vi "Full Density Matrix Heatmap.vi"(7 "QuWires Array":refnum<class "QuWire.lvclass">) -> ()   [LabVIEW 2020]
uses:
  QuSim/QuWire/QuWire.lvclass
panel:
  out "Real Amplitude":dbl[][](graph)
  out "Imaginary Amplltude":dbl[][](graph)
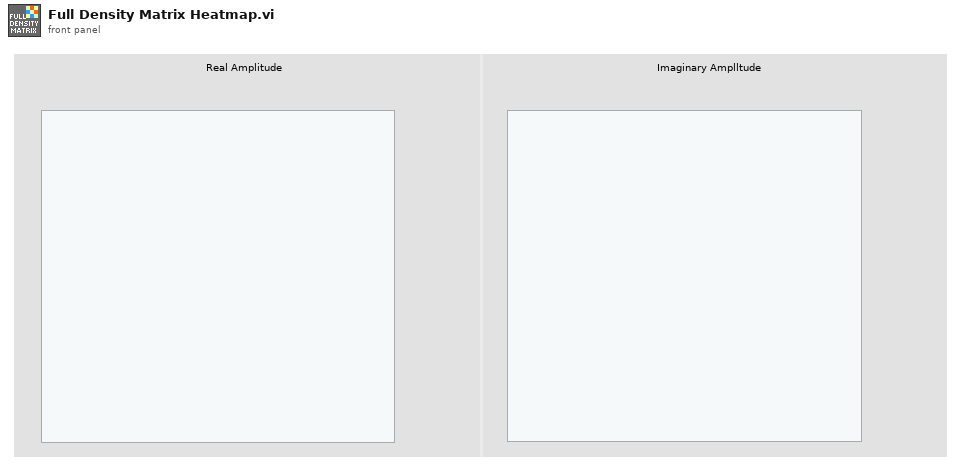
[diagram p1: front panel]
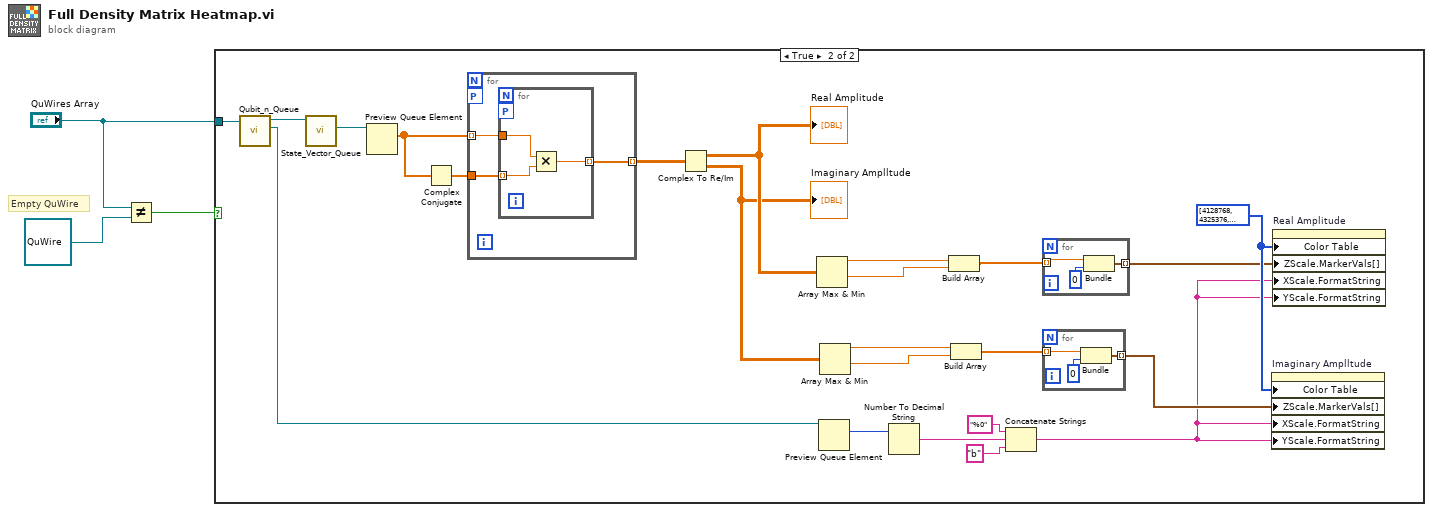
[diagram p0: block diagram]
diagram:
  # "Empty QuWire"
  n1 = Not Equal?(x="QuWires Array", y=refnum<class "QuWire.lvclass"> refnum ("QuWire in")) -> (x != y?=w1:bool)
  n2 = case shown="True" w1 {
    tunnel: "QuWires Array" -> [_ w7]
    frame False {
    }
    frame True {
      w26 = u32[] [4128768, 4325376, 4587520, 4718592, 4915200, 5111808, 5308416, 5505024, 5767168, 5963776, 6160384, 6356992, 6553600, 6750208, 6946816, 7143424, 7340032, 7536640, 7733248, 7929856, 8126464, 8323072, 8519680, 8716288, 8912896, 9109504, 9306112, 9502720, 9699328, 9895936, 10092544, 10289152, 10485760, 10682368, 10878976, 11075584, 11272192, 11468800, 11665408, 11862016, 12058624, 12255232, 12451840, 12648448, 12845056, 13041664, 13238272, 13434880, 13631488, 13828096, 14024704, 14221312, 14417920, 14614528, 14811136, 15007744, 15204352, 15400960, 15597568, 15794176, 16056320, 16187392, 16449536, 16580608, 16711937, 16647683, 16648453, 16649479, 16650250, 16585740, 16586510, 16587536, 16522770, 16523796, 16524566, 16460057, 16461083, 16396317, 16397343, 16398113, 16333604, 16334629, 16335400, 16270634, 16271660, 16272686, 16273713, 16208947, 16209716, 16210743, 16145977, 16147003, 16148029, 16083264, 16084290, 16019523, 16020806, 16021320, 16022602, 15957836, 15958607, 15959633, 15894867, 15896149, 15896663, 15832153, 15833179, 15834205, 15769440, 15770210, 15771236, 15706470, 15707496, 15708522, 15644012, 15644785, 15646076, 15712646, 15713936, 15715226, 15781797, 15783087, 15784377, 15850948, 15852238, 15853528, 15920098, 15921133, 15593455, 14871528, 14214882, 13558236, 12901845, 12179663, 11523016, 10866626, 10144444, 9487797, 8831407, 8109224, 7452578, 7189922, 7058595, 6927269, 6795687, 6664105, 6532778, 6466988, 6335407, 6204080, 6138290, 6006964, 5875382, 5744055, 5612729, 5481148, 5349821, 5283775, 5152449, 5021123, 4889540, 4823750, 4626888, 4560842, 4429516, 4298190, 4166608, 4035281, 3969491, 3837909, 3706583, 3575257, 3509211, 3312349, 3246303, 3114976, 2983650, 2852068, 2720742, 2654952, 2523370, 2392044, 2260717, 2194927, 1997809, 1932019, 1800693, 1669111, 1537785, 1406202, 1340412, 1209086, 1143038, 1142779, 1076728, 1076214, 1075699, 1075440, 1009134, 1008875, 1008360, 1007846, 941795, 941280, 941022, 874971, 874456, 873942, 873683, 807632, 807118, 806859, 806344, 740294, 739779, 739520, 739006, 672955, 672440, 672182, 606131, 605616, 605102, 604843, 538536, 538277, 537763, 537248, 471197, 470939, 470424, 469909, 403859, 403600, 403085, 337035, 336520, 336261, 335747, 269696, 269437, 268923, 268408, 202357, 202099, 201328, 135533, 135019, 134504, 133989, 67939, 67680, 67165, 66651, 600, 341] ("Color table")
      n3 = call "Qubit_n_Queue.vi"("QuWire in"=w7) -> ("Qubit n"=w5:refnum<queue>, "QuWire out"=w6:refnum<class "QuWire.lvclass">)  [unwired: 8 in, 1 out]
      n4 = call "State_Vector_Queue.vi"("QuWire in"=w6) -> ("State Vector Queue"=w11:refnum<queue>)  [unwired: 8 in, 2 out]
      n5 = Preview Queue Element(queue=w11) -> (element=w10:cdb[])  [unwired: 2 in, 3 out]
      n6 = Complex Conjugate(1:w10) -> (0:w9:cdb[])
      n7 = for {
        tunnel: w10 -> [w28] mode=indexing
        tunnel: w9 -> [w29]
        tunnel: [w27] -> w8 mode=indexing
        workers-P: _ -> [_]
        n8 = for {
          tunnel: w29 -> [w31] mode=indexing
          tunnel: w28 -> [w32]
          tunnel: [w30] -> w27 mode=indexing
          workers-P: _ -> [_]
          n9 = Multiply(x=w32, y=w31) -> (x*y=w30:cdb)
        }
      }
      n10 = Complex To Re/Im(x + iy=w8) -> (x=w23:dbl[][], y=w12:dbl[][])
      "Real Amplitude" <- w23
      "Imaginary Amplltude" <- w12
      n11 = Array Max & Min(array=w23) -> (max value=w24:dbl, min value=w25:dbl)  [unwired: 2 out]
      n12 = Preview Queue Element(queue=w5) -> (element=w4:i32)  [unwired: 2 in, 3 out]
      n13 = Array Max & Min(array=w12) -> (max value=w22:dbl, min value=w21:dbl)  [unwired: 2 out]
      n14 = Number To Decimal String(number=w4) -> (decimal integer string=w16:string)  [unwired: 1 in]
      n15 = Build Array(w24, w25) -> (w20:dbl[])
      n16 = Build Array(w22, w21) -> (w19:dbl[])
      n17 = Concatenate Strings("%0" ("string"), w16, "b" ("string")) -> (w13:string)
      n18 = for {
        tunnel: w20 -> [w38] mode=indexing
        tunnel: [w36] -> w18 mode=indexing
        n19 = Bundle(w38, 0) -> (w36:cluster{dbl, i32})  [unwired: 1 in]
      }
      n20 = for {
        tunnel: w19 -> [w35] mode=indexing
        tunnel: [w33] -> w17 mode=indexing
        n21 = Bundle(w35, 0) -> (w33:cluster{dbl, i32})  [unwired: 1 in]
      }
      n22 = property on="Imaginary Amplltude" class="IntGraph (strict)"("Color Table"=w26, "ZScale.MarkerVals[]"=w17, "XScale.FormatString"=w13, "YScale.FormatString"=w13) -> ()  [unwired: 2 in, 2 out]
      n23 = property on="Real Amplitude" class="IntGraph (strict)"("Color Table"=w26, "ZScale.MarkerVals[]"=w18, "XScale.FormatString"=w13, "YScale.FormatString"=w13) -> ()  [unwired: 2 in, 2 out]
    }
  }
